vi "convert-button-enum-to-cluster-of-booleans.vi"(11 "Controller button pressed enum":T1) -> (3 "Cluster":T2)   [LabVIEW 2020, in "GUI.lvlib"]
uses:
  GUI.lvlib
  Shared Ressources/Controller-button-pressed-enum.ctl
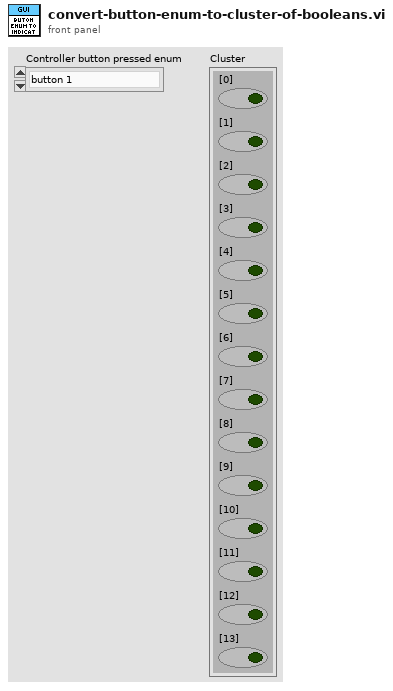
[diagram p1: front panel]
types:
  T1 = typedef "Controller-button-pressed-enum.ctl" = enum16{"button 1", "button 2", "button 3", "button 4", "button 5", "button 6", "button 7", "button 8", "button 9", "button 10", "button 11", "button 12", "button 13", "button 14"}
  T2 = cluster{"[0]":bool, "[1]":bool, "[2]":bool, "[3]":bool, "[4]":bool, "[5]":bool, "[6]":bool, "[7]":bool, "[8]":bool, "[9]":bool, "[10]":bool, "[11]":bool, "[12]":bool, "[13]":bool}
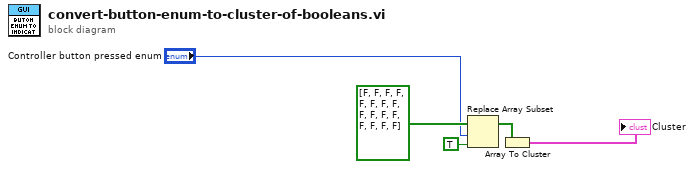
[diagram p0: block diagram]
diagram:
  n1 = Replace Array Subset(array=bool[] [FALSE, FALSE, FALSE, FALSE, FALSE, FALSE, FALSE, FALSE, FALSE, FALSE, FALSE, FALSE, FALSE, FALSE, FALSE, FALSE], new element=TRUE ("new element/subarray"), index="Controller button pressed enum") -> (w3:bool[])
  n2 = Array To Cluster(array=w3) -> (cluster=→"Cluster":T2)
